vi "IO.vi"() -> ()   [LabVIEW 2010]
panel:
  out "SMC Version":string
  out "Digital Output":bool[](array[boolean])
  out "Digital Input":bool[](array[boolean])
  out "Analog Input 1":dbl
  out "Analog Input 0":dbl
  in  "Analog Output 1 (set)":dbl=-3.25
  in  "Analog Output 0 (set)":dbl=7.0
  in  "Digital Output 1 (set)":i32=122 format="%02x"
  in  "Digital Output 0 (set)":i32=3 format="%01x"
  in  "Axis Name":string="X"
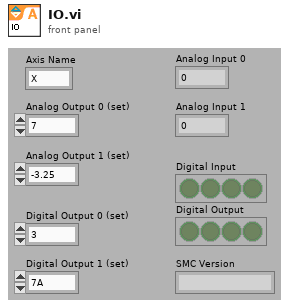
[diagram p1: front panel]
types:
  T1 = typedef "ControllerDiagPacket.ctl" = cluster{"Number of Diag Packets":i32, "Axes":T2[], "error":errorcluster}
  T2 = typedef "AxisDiagPacket.ctl" = cluster{"Axis Name":string, "Analog Input 0":dbl, "Analog Input 1":dbl, "Axis Fault (num)":i32, "Axis Fault (str)":string, "Axis Fault (bits)":cluster{"AmplifierFault":bool, "AmplifierTemperatureFault":bool, "CcwEndOfTravelLimitFault":bool, "CcwSoftwareLimitFault":bool, "CommunicationLostFault":bool, "CwEndOfTravelLimitFault":bool, "CwSoftwareLimitFault":bool, "EmergencyStopFault":bool, "EncoderFault":bool, "ExternalFault":bool, "FeedbackScalingFault":bool, "GantryMisalignFault ":bool, "HallSensorFault":bool, "InPositionTimeoutFault":bool, "InternalFault":bool, "MarkerSearchFault":bool, "MaxVelocityCommandFault":bool, "MissedInterruptFault":bool, "MotorTemperatureFault":bool, "None":bool, "OverCurrentFault":bool, "PositionErrorFault":bool, "PositionFeedbackFault":bool, "PowerSupplyFault":bool, "ProbeInputFault":bool, "SafeZoneFault":bool, "VelocityErrorFault":bool, "VelocityFeedbackFault":bool, "VoltageClampFault":bool}, "Axis Status (num)":i32, "Axis Status (str)":string, "Axis Status (bits)":cluster{"BacklashActive":bool, "CalibrationEnabled1D":bool, "CalibrationEnabled2D":bool, "CommandValid":bool, "DriveAbortPending":bool, "DrivePending":bool, "Enabling":bool, "GainMappingEnabled":bool, "GantryAligned":bool, "GantryRealigning":bool, "Homed":bool, "Homing":bool, "IFOVEnabled":bool, "JogGenerating":bool, "Jogging":bool, "JoystickControl":bool, "MasterSlaveControl":bool, "MotionBlocked":bool, "MotionClamped":bool, "MoveDone":bool, "None":bool, "NotVirtual":bool, "Profiling":bool, "Stability0":bool, "Stability1":bool, "TrajectoryFiltering":bool, "WaitDone":bool}, "Current Command":sgl, "Current Error":sgl, "Current Feedback":sgl, "Digital Inputs":i32, "Digital Outputs":i32, "Drive Status":i32, "Drive Status (str)":string, "Drive Status (bits)":cluster{"AccelerationPhase":bool, "AutofocusActive":bool, "BrakeOutput":bool, "CcwEndOfTravelLimitInput":bool, "CosineEncoderError":bool, "CurrentClamp":bool, "CwEndOfTravelLimitInput":bool, "DecelerationPhase":bool, "DualLoopActive":bool, "EmergencyStopInput":bool, "Enabled":bool, "EncoderClipping":bool, "GalvoCalibrationEnabled":bool, "GalvoPowerCorrection":bool, "HallAInput":bool, "HallBInput":bool, "HallCInput":bool, "HighResolutionMode":bool, "HomeLimitInput":bool, "InPosition":bool, "InPosition2":bool, "MarkerInput":bool, "MarkerLatch":bool, "MoveActive":bool, "NoMotorSupply":bool, "None":bool, "PowerLimiting":bool, "ProgrammingFlash":bool, "ProgrammingMXH":bool, "PSOHaltLatch":bool, "ServoControl":bool, "SineEncoderError":bool}, "Position Feedback Auxiliary":dbl, "Position Command":dbl, "Position Error":dbl, "Position Feedback":dbl, "Program Position Command":dbl, "Program Position Error":dbl, "Program Position Feedback":dbl, "Velocity Command":dbl, "Velocity Error":dbl, "Velocity Feedback":dbl}
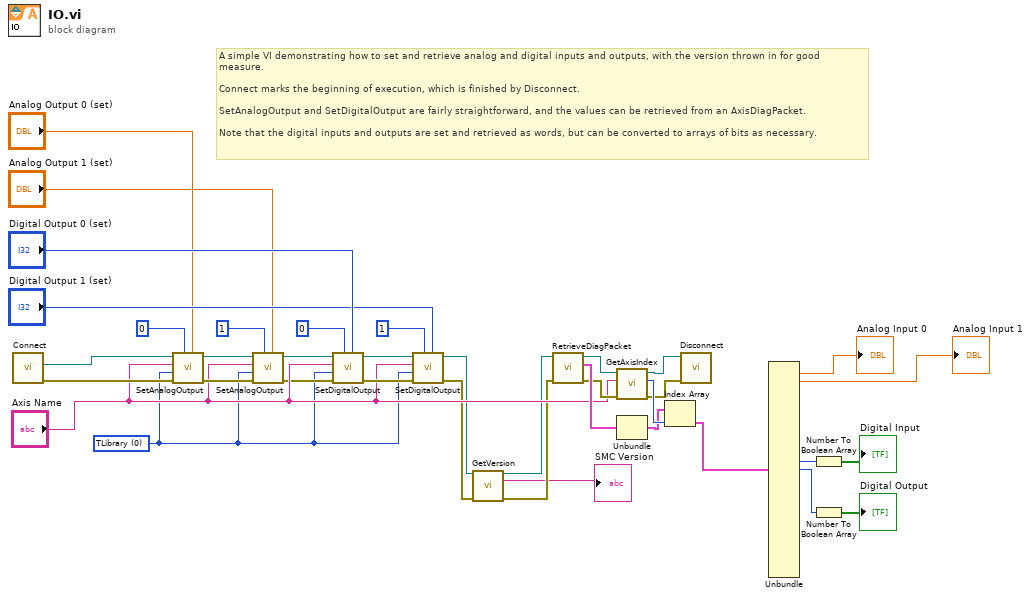
[diagram p0: block diagram]
diagram:
  w1 = 0 items=["TLibrary", "T01", "T02", "T03", "T04", "T05", "T06", "T07", "T08", "T09", "T10", "T11", "T12", "T13", "T14", "T15", "T16", "T17", "T18", "T19", "T20", "T21", "T22", "T23", "T24", "T25", "T26", "T27", "T28", "T29", "T30", "T31"] ("taskId")
  # "A simple VI demonstrating how to set and retrieve analog and digital inputs and outputs, with the version thrown in for good measure.\n\nConnect marks the beginning of execution, which is finished by Disconnect.\n\nSetAnalogOutput and SetDigitalOutput are fairly straightforward, and the values can be retrieved from an AxisDiagPacket.\n\nNote that the digital inputs and outputs are set and retrieved as words, but can be converted to arrays of bits as necessary."
  n1 = call "Connect.vi"() -> ("error out"=w24:errorcluster, "controller"=w25:refnum<k24>)  [unwired: 10 in]
  n2 = call "SetAnalogOutput.vi"("value"="Analog Output 0 (set)", "channel"=0 ("Port"), "error in (no error)"=w24, "taskId"=w1, "axis name"="Axis Name", "controller in"=w25) -> ("error out"=w22:errorcluster, "controller out"=w23:refnum<k24>)  [unwired: 4 in]
  n3 = call "SetAnalogOutput.vi"("value"="Analog Output 1 (set)", "channel"=1 ("Port"), "error in (no error)"=w22, "taskId"=w1, "axis name"="Axis Name", "controller in"=w23) -> ("error out"=w17:errorcluster, "controller out"=w18:refnum<k24>)  [unwired: 4 in]
  n4 = call "SetDigitalOutput.vi"("value"="Digital Output 0 (set)", "word"=0 ("Port"), "error in (no error)"=w17, "taskId"=w1, "axis name"="Axis Name", "controller in"=w18) -> ("error out"=w28:errorcluster, "controller out"=w29:refnum<k24>)  [unwired: 4 in]
  n5 = call "SetDigitalOutput.vi"("value"="Digital Output 1 (set)", "word"=1 ("Port"), "error in (no error)"=w28, "taskId"=w1, "axis name"="Axis Name", "controller in"=w29) -> ("error out"=w7:errorcluster, "controller out"=w6:refnum<k24>)  [unwired: 4 in]
  n6 = call "GetVersion.vi"("controller in"=w6, "error in (no error)"=w7) -> ("controller out"=w16:refnum<k24>, "SMC version"=→"SMC Version":string, "error out"=w15:errorcluster)  [unwired: 11 in]
  n7 = call "RetrieveDiagPacket.vi"("error in (no error)"=w15, "Controller In"=w16) -> ("error out"=w36:errorcluster, "ControllerDiagPacket"=w37:T1, "Controller Out"=w35:refnum<k24>)  [unwired: 7 in]
  n8 = call "GetAxisIndex.vi"("error in (no error)"=w36, "axis name"="Axis Name", "controller in"=w35) -> ("error out"=w30:errorcluster, "axis index"=w34:i32, "controller out"=w13:refnum<k24>)  [unwired: 6 in]
  n9 = Unbundle(w37) -> ("Axes"=w12:T2[])  [unwired: 2 out]
  n10 = Index Array(array=w12, index=w34) -> (element=w33:T2)
  n11 = call "Disconnect.vi"("error in (no error)"=w30, "controller"=w13) -> ()  [unwired: 9 in, 1 out]
  n12 = Unbundle(w33) -> ("Analog Input 0"=→"Analog Input 0":dbl, "Analog Input 1"=→"Analog Input 1":dbl, "Digital Inputs"=w9:i32, "Digital Outputs"=w8:i32)  [unwired: 23 out]
  n13 = Number To Boolean Array(number=w9) -> (Boolean array=→"Digital Input":bool[])
  n14 = Number To Boolean Array(number=w8) -> (Boolean array=→"Digital Output":bool[])
